vi "test - csm api path length.vi"(8 "error in (no error)":errorcluster, 11 "TestCase in":refnum<class "testcase-documentation.lvclass">) -> (0 "error out":errorcluster, 3 "TestCase out":refnum<class "testcase-documentation.lvclass">)   [LabVIEW 2017, in "testcase-documentation.lvclass"]
uses:
  testcase-documentation.lvclass
  <vilib>/addons/_JKI Toolkits/VI Tester/TestCase.llb/TestCase.lvclass
  src/user.lib/_NEVSTOP/Communicable State Machine(CSM)/Communicable State Machine.lvlib
  C:/Program Files (x86)/National Instruments/LabVIEW 2017/vi.lib/addons/_JKI Toolkits/VI Tester/TestCase.llb/TestCase.lvclass
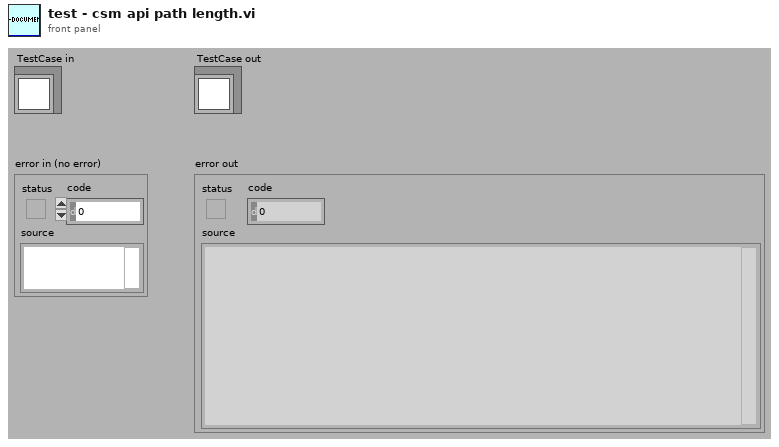
[diagram p1: front panel]
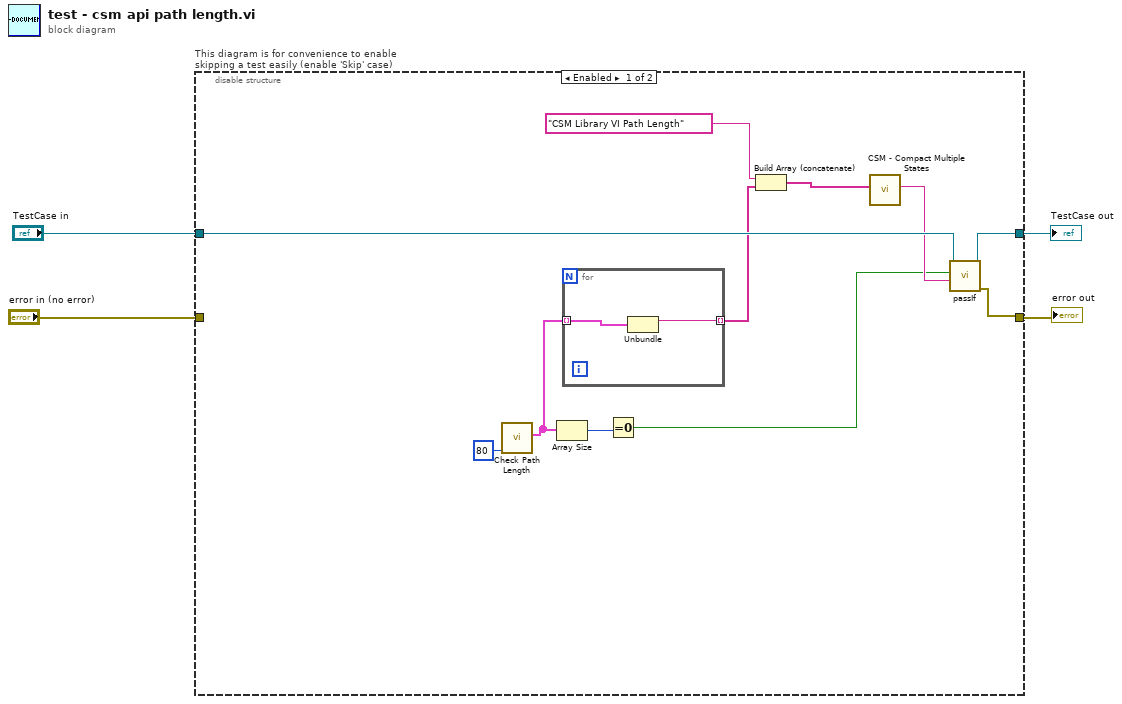
[diagram p0: block diagram]
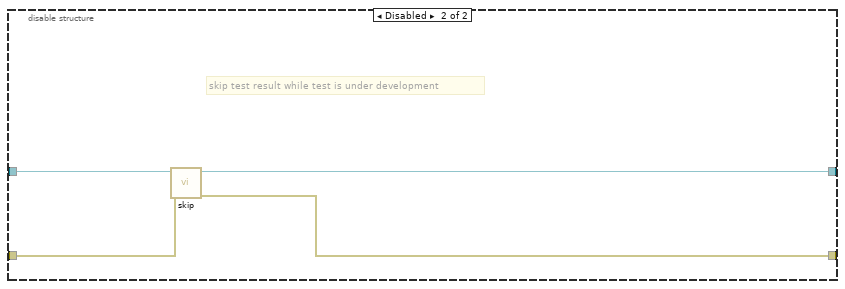
[diagram p2: hidden frame]
diagram:
  n1 = disable-structure "This diagram is for convenience to enable skipping a test easily (enable 'Skip' case)" shown="Enabled" {
    disable-tunnel: "TestCase in" -> [w15 w21]
    disable-tunnel: [w14 w19] -> w1
    disable-tunnel: [w13 w20] -> w3
    disable-tunnel: "error in (no error)" -> [_ w18]
    frame Enabled {
      n2 = call "Check Path Length.vi"("y"=80) -> ("Array"=w6:cluster{string, i32}[])  [unwired: 9 in, 1 out]
      n3 = Array Size(array=w6) -> (size(s)=w8:i32)
      n4 = for {
        tunnel: w6 -> [w17] mode=indexing
        tunnel: [w16] -> w5 mode=indexing
        n5 = Unbundle(w17) -> (w16:string)  [unwired: 1 out]
      }
      n6 = Equal To 0?(x=w8) -> (x = 0?=w7:bool)
      n7 = Build Array (concatenate)("CSM Library VI Path Length" ("message (\"\")"), w5) -> (w12:string[])
      n8 = call "CSM - Compact Multiple States.vi"("Multiple States"=w12) -> ("States"=w11:string)  [unwired: 9 in]
      n9 = call-dynamic "passIf.vi"("message (\"\")"=w11, "pass"=w7, "TestCase in"=w15) -> ("error out"=w13:errorcluster, "TestCase out"=w14:refnum<class "testcase-documentation.lvclass">)  [unwired: 7 in]
    }
    frame Disabled {
      # "skip test result while test is under development"
      n10 = call <vilib>:"skip.vi"("error in (no error)"=w18, "TestCase in"=w21) -> ("error out"=w20:errorcluster, "TestCase out"=w19:refnum<class "testcase-documentation.lvclass">)  [unwired: 8 in]
    }
  }
  "error out" <- w3
  "TestCase out" <- w1
